vi "mmap.vi"(6 "process (shared)":T1, 7 "protections (read/write)":T2={"read"=TRUE, "write"=TRUE, "execute"=FALSE}, 8 "error in (no error)":errorcluster, 9 "offset (0)":u64, 10 "number of bytes":u64, 11 "file descriptor":i32) -> (0 "error out":errorcluster, 2 "pointer":u64 format="0x%016x", 3 "file descriptor":i32)   [LabVIEW 2016, in "Linux RT IPC.C.lvlib"]
doc: "Wrapper VI for Linux function mmap()."
uses:
  Linux RT IPC.C.lvlib
  Controls/mman sharing.ctl
  Controls/functions.ctl
  <vilib>/NI/NI Linux RT Errno/Linux Errno.lvlib
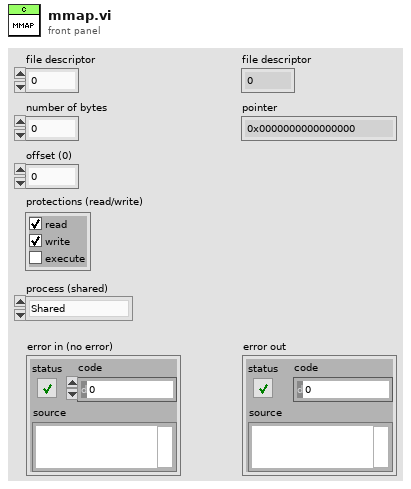
[diagram p1: front panel]
types:
  T1 = typedef "Linux RT IPC.C.lvlib/mman sharing.ctl" = enum16{"Shared", "Private"}
  T2 = cluster{"read":bool, "write":bool, "execute":bool}
  T3 = typedef "Linux RT IPC.C.lvlib/functions.ctl" = enum16{"unspecified", "close", "epoll_create", "epoll_ctl", "epoll_wait", "fstat", "ftruncate", "mkfifo", "mmap", "munmap", "open", "read", "shm_open", "shm_unlink", "timerfd_create", "timerfd_settime", "timerfd_gettime", "write", "unlink"}
  T4 = typedef "Linux Errno.lvlib/errno.ctl" = enum16{"NO ERROR", "EPERM", "ENOENT", "ESRCH", "EINTR", "EIO", "ENXIO", "E2BIG", "ENOEXEC", "EBADF", "ECHILD", "EAGAIN", "ENOMEM", "EACCES", "EFAULT", "ENOTBLK", "EBUSY", "EEXIST", "EXDEV", "ENODEV", "ENOTDIR", "EISDIR", "EINVAL", "ENFILE", "EMFILE", "ENOTTY", "ETXTBSY", "EFBIG", "ENOSPC", "ESPIPE", "EROFS", "EMLINK", "EPIPE", "EDOM", "ERANGE", "EDADLK", "ENAMETOOLONG", "ENOLCK", "ENOSYS", "ENOTEMPTY", "ELOOP", "EWOULDBLOCK", "ENOMSG", "EIDRM", "ECHRNG", "EL2NSYNC", "EL3HLT", "EL3RST", "ELNRNG", "EUNATCH", "ENOCSI", "EL2HLT", "EBADE", "EBADR", "EXFULL", "ENOANO", "EBADRQC", "EBADSLT", "EDEADLOCK", "EBFONT", "ENOSTR", "ENODATA", "ETIME", "ENOSR", "ENONET", "ENOPKG", "EREMOTE", "ENOLINK", "EADV", "ESRMNT", "ECOMM", "EPROTO", "EMULTIHOP", "EDOTDOT", "EBADMSG", "EOVERFLOW", "ENOTUNIQ", "EBADFD", "EREMCHG", "ELIBACC", "ELIBBAD", "ELIBSCN", "ELIBMAX", "ELIBEXEC", "ELISEQ", "ERESTART", "ESTRPIPE", "EUSERS", "ENOTSOCK", "EDESTADDRREQ", "EMSGSIZE", "EPROTOTYPE", "ENOPROTOOPT", "EPROTONOSUPPORT", "ESOCKTNOSUPPORT", "EOPNOTSUPP", "EPFNOSUPPORT", "EAFNOSUPPORT", "EADDRINUSE", "EADDRNOTAVAIL", "ENETDOWN", "ENETUNREACH", "ENETRESET", "ECONNABORTED", "ECONNRESET", "ENOBUFS", "EISCONN", "ENOTCONN", "ESHUTDOWN", "ETOOMANYREFS", "ETIMEDOUT", "ECONNREFUSED", "EHOSTDOWN", "EHOSTUNREACH", "EALREADY", "EINPROGRESS", "ESTALE", "EUCLEAN", "ENOTNAM", "ENAVAIL", "EISNAM", "EREMOTEIO", "EDQUOT", "ENOMEDIUM", "EMEDIUMTYPE", "ECANCELED", "ENOKEY", "EKEYEXPIRED", "EKEYREVOKED", "EKEYREJECTED", "EOWNERDEAD", "ENOTRECOVERABLE", "ERFKILL", "EHWPOISON", "UNDEFINED"}
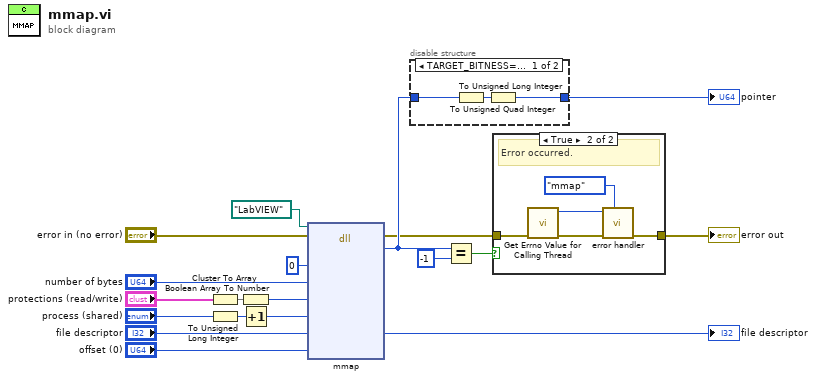
[diagram p0: block diagram]
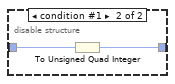
[diagram p3: hidden frame]
diagram:
  n1 = Cluster To Array(cluster="protections (read/write)") -> (array=w10:bool[])
  n2 = To Unsigned Long Integer(number="process (shared)") -> (unsigned 32bit integer=w9:u32)
  n3 = Boolean Array To Number(Boolean array=w10) -> (number=w7:u32)
  n4 = Increment(x=w9) -> (x+1=w6:u32)
  n5 = dll-call lib="?" fn="mmap"(path in=path "LabVIEW", error in="error in (no error)", "addr"=u64 0, "size"="number of bytes", "prot"=w7, "flags"=w6, "fd"="file descriptor", "offset"="offset (0)") -> (error out=w3:errorcluster, "pointer"=w4:i64, "fd"=→"file descriptor":i32)  [unwired: 6 in, 1 out]
  n6 = disable-structure shown="TARGET_BITNESS==32" {
    disable-tunnel: w4 -> [w20 w24]
    disable-tunnel: [w22 w23] -> w14
    frame condition #0 (active) {
      n7 = To Unsigned Long Integer(number=w20) -> (unsigned 32bit integer=w21:u32)
      n8 = To Unsigned Quad Integer(1:w21) -> (0:w22:u64)
    }
    frame condition #1 {
      n9 = To Unsigned Quad Integer(1:w24) -> (0:w23:u64)
    }
  }
  "pointer" <- w14
  n10 = Equal?(x=w4, y=i64 -1) -> (x = y?=w2:bool)
  n11 = case shown="True" w2 {
    tunnel: w3 -> [w25 w30]
    tunnel: [w25 w28] -> w18
    frame False {
      # "No error."
    }
    frame True {
      # "Error occurred."
      n12 = call <vilib>:"Get Errno Value for Calling Thread.vi"("error in (no error)"=w30) -> ("error out"=w29:errorcluster, "errno"=w27:T4)  [unwired: 9 in]
      n13 = call "error handler.vi"("function (unspecified)"=functions."mmap", "error in (no error)"=w29, "errno"=w27) -> ("error out"=w28:errorcluster)  [unwired: 8 in]
    }
  }
  "error out" <- w18
